vi "get hydrolysis PH.vi"(8 "error in (no error)":errorcluster, 10 "reactor_state_files":string) -> (0 "error out":errorcluster, 2 "ph_string":string)   [LabVIEW 2019, in "libFileFunctions.lvlib"]
doc: "void get_hydrolysis_PH(double (&ph_arr)[3], const char* reactor_state_files);"
uses:
  libFileFunctions.lvlib
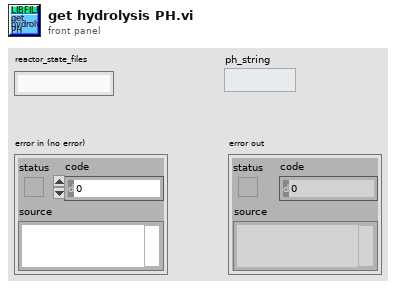
[diagram p1: front panel]
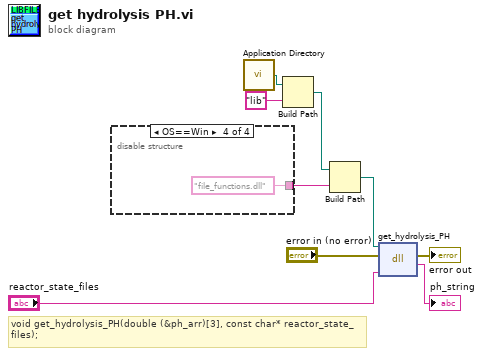
[diagram p0: block diagram]
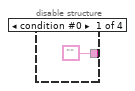
[diagram p2: hidden frame]
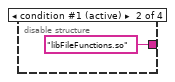
[diagram p3: hidden frame]
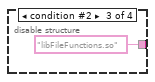
[diagram p4: hidden frame]
diagram:
  # "void get_hydrolysis_PH(double (&ph_arr)[3], const char* reactor_state_files);"
  n1 = disable-structure shown="OS==Win" {
    disable-tunnel: ["" "libFileFunctions.so" ("name or relative path") "libFileFunctions.so" ("name or relative path") "file_functions.dll" ("name or relative path")] -> w3
    frame condition #0 {
    }
    frame condition #1 (active) {
    }
    frame condition #2 {
    }
    frame condition #3 {
    }
  }
  n2 = call <vilib>:"Application Directory.vi"() -> ("Application Directory"=w6:path)
  n3 = Build Path(base path=w6, name or relative path="lib") -> (appended path=w4:path)
  n4 = Build Path(base path=w4, name or relative path=w3) -> (appended path=w2:path)
  n5 = dll-call lib="home/paul/Schreibtisch/Biogas_plant_setup/LabView/lib/libFileFunctions/libFileFunctions.*" fn="get_hydrolysis_PH"(path in=w2, error in="error in (no error)", "reactor_state_files"="reactor_state_files") -> (error out=→"error out":errorcluster, "ph_string"=→"ph_string":string)  [unwired: 2 in, 1 out]
